vi "EtherCAT Connection Updated.vi"(8 "error in":errorcluster, 10 "Connection Status":bool) -> (0 "error out":errorcluster)   [LabVIEW 2024, in "EtherCAT Model.lvlib"]
doc: "This broadcast lets modules know that the connection status of the ethercat has changed\n_____\nCreated using DQMH Event Scripter 7.0.0.1280."
uses:
  EtherCAT Model.lvlib
  EtherCAT Connection Updated Argument--cluster.ctl
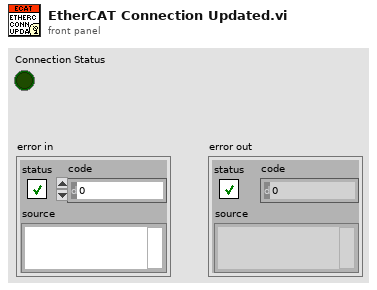
[diagram p1: front panel]
types:
  T1 = typedef "EtherCAT Model.lvlib/EtherCAT Connection Updated Argument--cluster.ctl" = cluster{"Connection Status":bool}
  T2 = typedef "EtherCAT Model.lvlib/Broadcast Events--cluster.ctl" = cluster{"Module Did Init":refnum<user-event>, "Status Updated":refnum<user-event>, "Error Reported":refnum<user-event>, "Module Did Stop":refnum<user-event>, "Update Module Execution Status":refnum<user-event>, "Raw Data Updated":refnum<user-event>, "Date Updated":refnum<user-event>, "EtherCAT Connection Updated":refnum<user-event>}
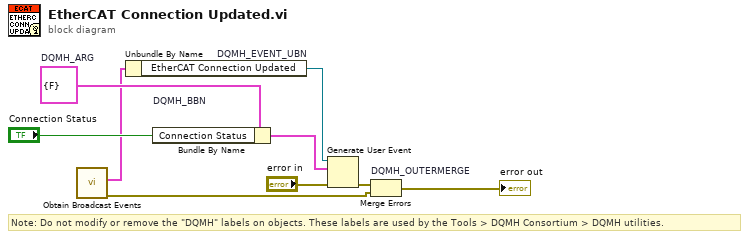
[diagram p0: block diagram]
diagram:
  w4 = T1 {"Connection Status"=FALSE}  # DQMH_ARG
  # "Note: Do not modify or remove the \"DQMH\" labels on objects. These labels are used by the Tools > DQMH Consortium > DQMH utilities."
  n1 = call "Obtain Broadcast Events.vi"() -> ("error out"=w2:errorcluster, "EtherCAT Model Broadcast Events"=w1:T2)  [unwired: 10 in]
  n2 = Unbundle By Name "DQMH_EVENT_UBN"(w1) -> ("EtherCAT Connection Updated"=w6:refnum<user-event>)
  n3 = Bundle By Name "DQMH_BBN"(cluster=w4, "Connection Status"="Connection Status") -> (w7:T1)
  n4 = Generate User Event(user event=w6, event data cluster=w7, error in="error in") -> (error out=w5:errorcluster)  [unwired: 1 in, 1 out]
  n5 = Merge Errors "DQMH_OUTERMERGE"(w5, w2) -> (→"error out":errorcluster)
